vi "Emballage_BDD_Choix_Config_initListe.vi"(8 "entrée d'erreur (pas d'erreur)":errorcluster, 10 "where valeur":string[](array[string]), 11 "Where colonne":string[](array[string])) -> (0 "sortie d'erreur":errorcluster, 3 "chemin complet":path)   [LabVIEW 2020]
uses:
  <vilib>/Utility/miscctls.llb/LVRowAndColumnUnsignedTypeDef.ctl
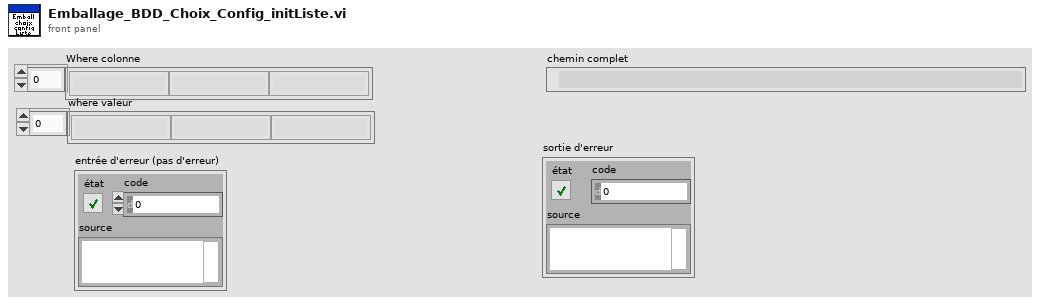
[diagram p1: front panel]
types:
  T1 = typedef "LVRowAndColumnUnsignedTypeDef.ctl" = cluster{"Row":u32, "Column":u32}
  T2 = typedef "Choix_Config_ref.ctl" = cluster{"No_Valve_FAS":refnum<vi>, "Liste multicolonne":refnum<vi>, "suffixe":refnum<vi>, "designation":refnum<vi>, "Famille":refnum<vi>}
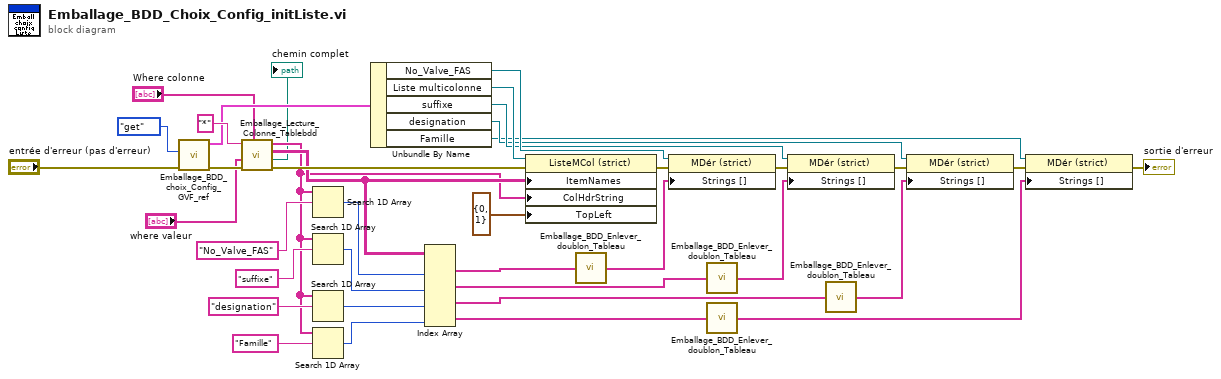
[diagram p0: block diagram]
diagram:
  n1 = call "Emballage_BDD_choix_Config_GVF_ref.vi"("Error in"="entrée d'erreur (pas d'erreur)", "Énum"=enum16{"get", "set"}."get") -> ("Error out"=w6:errorcluster, "Cluster OUT"=w13:T2)  [unwired: 8 in]
  n2 = call "Emballage_Lecture_Colonne_Tablebdd.vi"("Where colonne"="Where colonne", "Error in"=w6, "where valeur"="where valeur", "Colonne"="*") -> ("Error out"=w33:errorcluster, "chemin complet"=→"chemin complet":path, "Result Set"=w16:string[][], "Column Names"=w4:string[])  [unwired: 4 in]
  n3 = Search 1D Array(1D array=w4, element="No_Valve_FAS" ("élément")) -> (index of element=w18:i32)  [unwired: 1 in]
  n4 = Search 1D Array(1D array=w4, element="suffixe" ("élément")) -> (index of element=w20:i32)  [unwired: 1 in]
  n5 = Search 1D Array(1D array=w4, element="designation" ("élément")) -> (index of element=w22:i32)  [unwired: 1 in]
  n6 = Search 1D Array(1D array=w4, element="Famille" ("élément")) -> (index of element=w24:i32)  [unwired: 1 in]
  n7 = Unbundle By Name(w13) -> ("No_Valve_FAS"=w11:refnum<vi>, "Liste multicolonne"=w12:refnum<vi>, "suffixe"=w10:refnum<vi>, "designation"=w9:refnum<vi>, "Famille"=w8:refnum<vi>)
  n8 = Index Array(array=w16, index (col) #1=w18, index (col) #2=w20, index (col) #3=w22, index (col) #4=w24) -> (element #1=w25:string[], element #2=w31:string[], element #3=w29:string[], element #4=w27:string[])  [unwired: 4 in]
  n9 = property on="Nœud de propriété" class="ListeMCol (strict)"(reference=w12, error in=w33, "ItemNames"=w16, "ColHdrString"=w4, "TopLeft"=T1 {"Row"=0, "Column"=1} ("Cellule visible en haut à gauche")) -> (error out=w34:errorcluster)  [unwired: 1 out]
  n10 = call "Emballage_BDD_Enlever_doublon_Tableau.vi"("Tableau_IN"=w25) -> ("Tableau_OUT"=w26:string[])
  n11 = property on="Nœud de propriété" class="MDér (strict)"(reference=w11, error in=w34, "Strings []"=w26) -> (error out=w35:errorcluster)  [unwired: 1 out]
  n12 = call "Emballage_BDD_Enlever_doublon_Tableau.vi"("Tableau_IN"=w31) -> ("Tableau_OUT"=w32:string[])
  n13 = call "Emballage_BDD_Enlever_doublon_Tableau.vi"("Tableau_IN"=w27) -> ("Tableau_OUT"=w28:string[])
  n14 = property on="Nœud de propriété" class="MDér (strict)"(reference=w10, error in=w35, "Strings []"=w32) -> (error out=w36:errorcluster)  [unwired: 1 out]
  n15 = call "Emballage_BDD_Enlever_doublon_Tableau.vi"("Tableau_IN"=w29) -> ("Tableau_OUT"=w30:string[])
  n16 = property on="Nœud de propriété" class="MDér (strict)"(reference=w9, error in=w36, "Strings []"=w30) -> (error out=w37:errorcluster)  [unwired: 1 out]
  n17 = property on="Nœud de propriété" class="MDér (strict)"(reference=w8, error in=w37, "Strings []"=w28) -> (error out=→"sortie d'erreur":errorcluster)  [unwired: 1 out]
